vi "Wrapper.vi"(8 "error in":errorcluster, 10 "Controller in in":refnum<class "Controller.lvclass">, 11 "Change Filter State MSG in":refnum<class "Change Filter State.lvclass">) -> (0 "error out":errorcluster, 3 "Controller out":refnum<class "Controller.lvclass">)   [LabVIEW 2014, in "Controller.lvlib" / "Change Filter State.lvclass"]
uses:
  Change Filter State.lvclass
  Controller.lvclass
  Controls/Enqueuer Enum.ctl
  CRDS/Actor Messages/Change Filter State/Change Filter State.lvclass
  PAS/Actor/Messages/Update Filter MSG/Change Filter State.lvclass
  Update Switch State MSG/Update Switch MSG.lvclass/Update Switch MSG.ctl
  SuperActor/SuperActor.lvclass/SuperActor.ctl
  Controller.lvclass/Controller.ctl
  PAS/Actor/Messages/Update Filter MSG/Change Filter State.lvclass/Change Filter State.ctl
  CRDS/Actor Messages/Change Filter State/Change Filter State.lvclass/Change Filter State.ctl
  Controls/eMap.ctl
  <vilib>/ActorFramework/Message Enqueuer/Message Enqueuer.lvclass
  Instr Actor/Messages/Change Speaker State/Change Speaker Switch MSG.lvclass
  <vilib>/ActorFramework/Message Enqueuer/Message Enqueuer.lvclass/Message Enqueuer.ctl
  Update Switch State MSG/Write SwitchState.vi
  Update Switch State MSG/Read SwitchState.vi
  SuperActor/Read CVT Session.vi
  SuperActor/Read Log Session.vi
  Accessors/Read Switch DVR.vi
  <vilib>/ActorFramework/Message Priority Queue/Priority Enqueue.vi
  <vilib>/DAQmx/write.llb/DAQmx Write (Digital 1D Bool NChan 1Samp 1Line).vi
  <vilib>/DAQmx/write.llb/DAQmx Write (Digital Bool 1Line 1Point).vi
  <userlib>/_Session Fwk/Session - Root.lvclass
  reusable/Switch/Switch.lvclass
  reusable/Session APIs/Session Log/System Log.lvclass
  reusable/Session APIs/CVT/CVT.lvclass
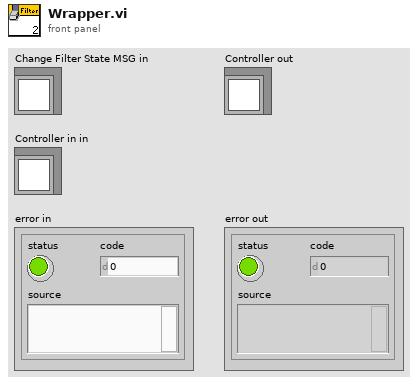
[diagram p1: front panel]
types:
  T1 = typedef "Controller.lvlib/Controller.lvclass/Enqueuer Enum.ctl" = enum8{"PAS", "CRDS", "File", "O3Lamp"}
  T2 = typedef "Session - Root.lvclass/Session Handle.ctl" = refnum<data-value>
  T3 = typedef "Controller.lvlib/Controller.lvclass/eMap.ctl" = cluster{"Enqueuer":refnum<class "Message Enqueuer.lvclass">, "Active":bool}
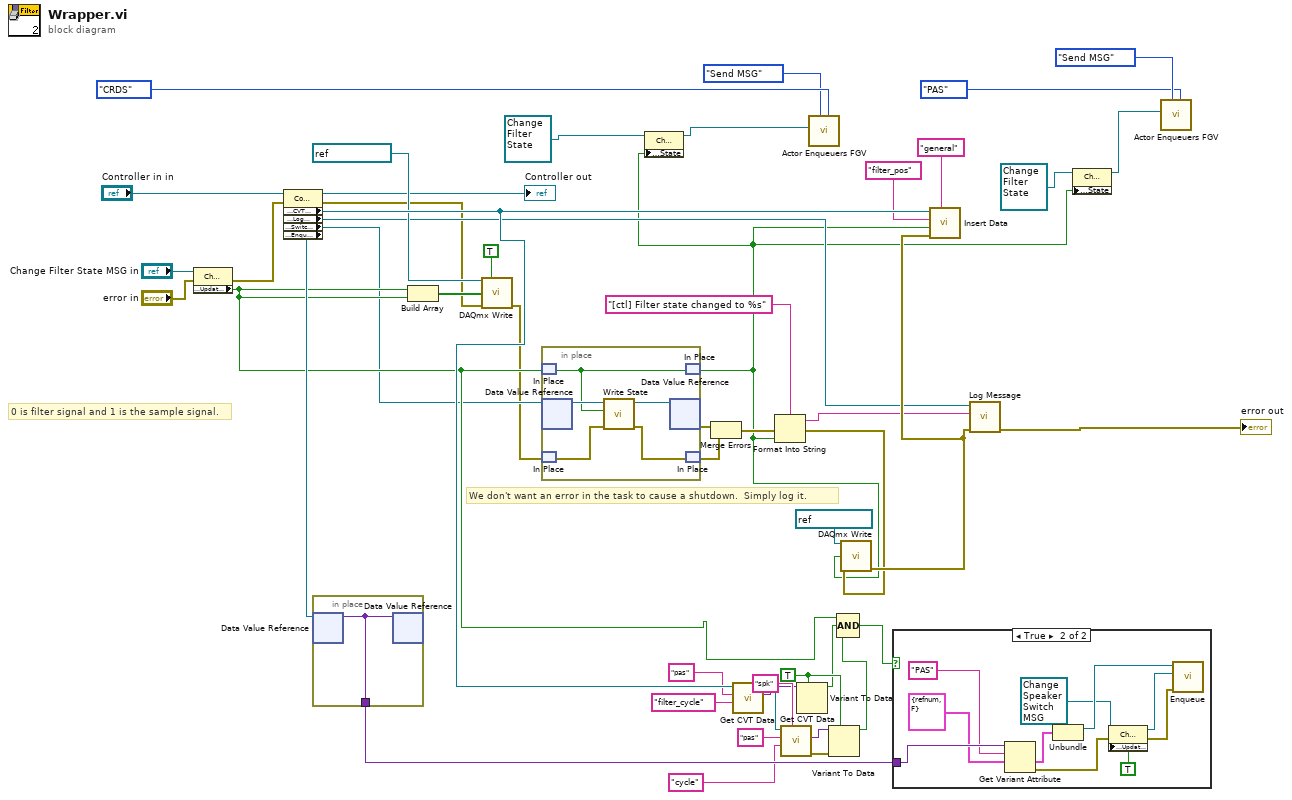
[diagram p0: block diagram]
diagram:
  w40 = TRUE
  # "0 is filter signal and 1 is the sample signal."
  # "We don't want an error in the task to cause a shutdown.  Simply log it."
  n1 = property class="Change Filter State MSG"(reference="Change Filter State MSG in", error in="error in") -> (error out=w28:errorcluster, "Accessors:UpdateSw"=w43:bool)  [unwired: 1 out]
  n2 = property class="Controller"(reference="Controller in in", error in=w28) -> (reference out=→"Controller out":refnum<class "Controller.lvclass">, error out=w15:errorcluster, "Accessors:CVT Session"=w44:T2, "Accessors:Log Session"=w19:T2, "Accessors:Switch DVR"=w23:refnum<data-value>, "Accessors:Enqueuer MAP DVR"=w45:refnum<data-value>)
  n3 = in-place {
    in-place-border: [w50] -> w46
    n4 = in-place-dvr #1(w45) -> (w50:variant)  [unwired: 1 out]
    n5 = in-place-dvr #1(w50) -> ()  [unwired: 2 out]
  }
  n6 = Build Array(w43, w43) -> (w16:bool[])
  n7 = call-poly <vilib>:"DAQmx Write.vi"("task/channels in"=refnum<k21> "Filter Valve CMD", "auto start"=TRUE, "data"=w16, "error in"=w15) -> ("error out"=w21:errorcluster)  [unwired: 9 in, 2 out]
  n8 = in-place {
    n9 = in-place-match #2(w43) -> (w51:bool)
    n10 = in-place-dvr #3(w23) -> (w55:refnum<class "Switch.lvclass">)  [unwired: 1 out]
    n11 = in-place-match #4(w21) -> (w52:errorcluster)
    n12 = call-dynamic "Write State.vi"("error in"=w52, "State"=w51, "Switch in"=w55) -> ("error out"=w53:errorcluster, "Switch out"=w54:refnum<class "Switch.lvclass">)  [unwired: 7 in]
    n13 = in-place-dvr #3(w54) -> (w11:errorcluster)  [unwired: 1 out]
    n14 = in-place-match #2(w51) -> (w2:bool)
    n15 = in-place-match #4(w53) -> (w20:errorcluster)
  }
  n16 = property class="Change Filter State.lvclass"(reference=refnum<class "Change Filter State.lvclass"> refnum ("eCRDS Library.lvlib:Change Filter State.lvclass"), "Accessors:State"=w2) -> (reference out=w7:refnum<class "Change Filter State.lvclass">)  [unwired: 1 in, 1 out]
  n17 = Merge Errors(w11, w20) -> (w22:errorcluster)
  n18 = call "Get CVT Data.vi"("Variable"="filter_cycle", "Group"="pas" ("Subgroup"), "CVT Session In"=w44) -> ("Data Out"=w32:variant, "CVT Session Out"=w35:T2)  [unwired: 5 in, 2 out]
  n19 = Format Into String(format string="[ctl] Filter state changed to %s" ("MSG In"), error in=w22, w2) -> (resulting string=w14:string, error out=w48:errorcluster)  [unwired: 1 in]
  n20 = call "Get CVT Data.vi"("Subgroup"="spk", "Variable"="cycle" ("Group"), "Group"="pas", "CVT Session In"=w35) -> ("error out"=w38:errorcluster, "Data Out"=w39:variant)  [unwired: 4 in, 2 out]
  n21 = Variant To Data(type=w40, Variant=w32) -> (data=w33:bool)  [unwired: 1 in, 1 out]
  n22 = call "Actor Enqueuers FGV.vi"("Enqueuer"=Enqueuer_Enum."CRDS", "State"=enum16{"Store", "Send MSG"}."Send MSG", "MSG"=w7) -> ()  [unwired: 8 in, 1 out]
  n23 = Variant To Data(error in=w38, type=w40, Variant=w39) -> (data=w41:bool)  [unwired: 1 out]
  n24 = Compound Arithmetic op=AND(w43, w33, w41) -> (w34:bool)
  n25 = call-poly <vilib>:"DAQmx Write.vi"("task/channels in"=refnum<k21> "Filter LED", "data"=w2, "error in"=w48) -> ("error out"=w49:errorcluster)  [unwired: 10 in, 2 out]
  n26 = case shown="True" w34 {
    tunnel: w46 -> [_ w65]
    frame False {
    }
    frame True {
      n27 = Get Variant Attribute(Variant=w65, name="PAS", default value (empty Variant)=T3 {"Enqueuer"=refnum, "Active"=FALSE} ("eMap")) -> (value=w62:T3, error out=w57:errorcluster)  [unwired: 1 in, 2 out]
      n28 = Unbundle(w62) -> ("Enqueuer"=w61:refnum<class "Message Enqueuer.lvclass">)  [unwired: 1 out]
      n29 = property class="Change Speaker MSG"(reference=refnum<class "Change Speaker Switch MSG.lvclass"> refnum ("ePAS Library.lvlib:Change Speaker MSG"), error in=w57, "Accessors:UpdateSw"=TRUE ("UpdateSw")) -> (reference out=w58:refnum<class "Change Speaker Switch MSG.lvclass">, error out=w56:errorcluster)
      n30 = call <vilib>:"Enqueue.vi"("error in (no error)"=w56, "Message"=w58, "Message Enqueuer in"=w61) -> ()  [unwired: 7 in, 2 out]
    }
  }
  n31 = call "Insert Data.vi"("Group"="general", "error in"=w49, "Data"=w2, "tag"="filter_pos", "CVT Session In"=w44) -> ()  [unwired: 5 in, 2 out]
  n32 = call "Log Message.vi"("error in"=w49, "MSG In"=w14, "session in"=w19) -> ("error out"=→"error out":errorcluster)  [unwired: 7 in, 1 out]
  n33 = property class="Change Filter State.lvclass"(reference=refnum<class "Change Filter State.lvclass"> refnum ("ePAS Library.lvlib:Change Filter State.lvclass"), "Accessors:State"=w2) -> (reference out=w1:refnum<class "Change Filter State.lvclass">)  [unwired: 1 in, 1 out]
  n34 = call "Actor Enqueuers FGV.vi"("Enqueuer"=Enqueuer_Enum."PAS", "State"=enum16{"Store", "Send MSG"}."Send MSG", "MSG"=w1) -> ()  [unwired: 8 in, 1 out]
